vi "BouncingBall.vi"() -> ()   [LabVIEW 2024]
uses:
  <vilib>/picture/3D Picture Control/Object/Create Object (drawable).vi
  <vilib>/picture/3D Picture Control/NI_3D Picture Control.lvlib
panel:
  out "3D Picture":refnum<vi>(3d-picture)
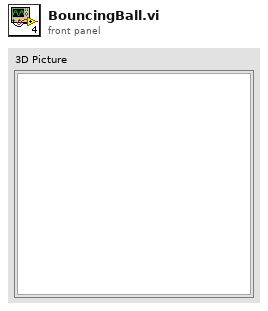
[diagram p1: front panel]
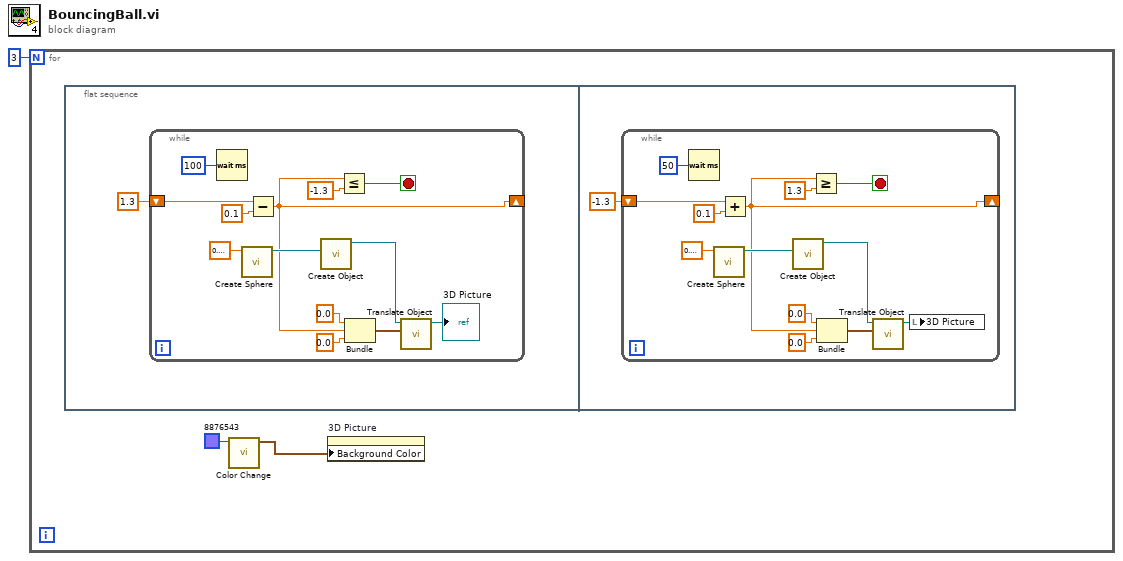
[diagram p0: block diagram]
diagram:
  n1 = for {
    N: 3 -> [_]
    n2 = flat-sequence {
      frame #0 {
        n3 = while {
          shift-right: [w8] -> _
          shift-left: 1.3 -> [w11]
          stop <- w9 stop-if-true
          n4 = Wait (ms)(milliseconds to wait=u32 100) -> ()  [unwired: 1 out]
          n5 = call <vilib>:"Create Sphere.vi"("Radius"=sgl 0.3) -> ("New Sphere Refnum"=w17:refnum<vi>)  [unwired: 9 in, 1 out]
          n6 = Subtract(x=w11, y=0.1) -> (x-y=w8:dbl)
          n7 = call-poly <vilib>:"Create Object.vi"("Geometry"=w17) -> ("Scene:New Object"=w15:refnum<vi>)  [unwired: 9 in, 1 out]
          n8 = Less Or Equal?(x=w8, y=-1.3) -> (x <= y?=w9:bool)
          n9 = Bundle(0.0, w8, 0.0) -> (w7:cluster{dbl, dbl, dbl})  [unwired: 1 in]
          n10 = call <vilib>:"Translate Object.vi"("Translation"=w7, "Scene.Object In"=w15) -> ("Scene.Object Out"=→"3D Picture":refnum<vi>)  [unwired: 8 in, 1 out]
        }
      }
      frame #1 {
        n11 = while {
          shift-right: [w22] -> _
          shift-left: -1.3 -> [w25]
          stop <- w23 stop-if-true
          n12 = Wait (ms)(milliseconds to wait=u32 50) -> ()  [unwired: 1 out]
          n13 = call <vilib>:"Create Sphere.vi"("Radius"=sgl 0.3) -> ("New Sphere Refnum"=w31:refnum<vi>)  [unwired: 9 in, 1 out]
          n14 = Add(x=w25, y=0.1) -> (x+y=w22:dbl)
          n15 = call-poly <vilib>:"Create Object.vi"("Geometry"=w31) -> ("Scene:New Object"=w29:refnum<vi>)  [unwired: 9 in, 1 out]
          n16 = Greater Or Equal?(x=w22, y=1.3) -> (x >= y?=w23:bool)
          n17 = Bundle(0.0, w22, 0.0) -> (w21:cluster{dbl, dbl, dbl})  [unwired: 1 in]
          n18 = call <vilib>:"Translate Object.vi"("Translation"=w21, "Scene.Object In"=w29) -> ("Scene.Object Out"=w19:refnum<vi>)  [unwired: 8 in, 1 out]
          n19 = local write "3D Picture"(w19) -> ()
        }
      }
    }
    n20 = call <vilib>:"Color Change.vi"("Color"=u32 8876543) -> ("RGBA"=w3:cluster{"R":sgl, "G":sgl, "B":sgl, "A":sgl})  [unwired: 10 in]
    n21 = property on="3D Picture" class="SceneGraphDisp (strict)"("Background Color"=w3) -> ()  [unwired: 2 in, 2 out]
  }
